vi "Save.vi"(0 "Reporte IN":refnum<class "NI_report.lvclass">, 7 "Error IN":errorcluster, 8 "X1":dbl[](array[numeric]), 9 "X7":dbl[](array[numeric]), 10 "X2":dbl[](array[numeric]), 11 "X8":dbl[](array[numeric]), 12 "X3":dbl[](array[numeric]), 13 "X9":dbl[](array[numeric]), 14 "X4":dbl[](array[numeric]), 16 "X5":dbl[](array[numeric]), 18 "X6":dbl[](array[numeric])) -> (20 "Reporte Out":refnum<class "NI_report.lvclass">, 27 "ERROR OUT":errorcluster)   [LabVIEW 2021]
uses:
  <vilib>/Utility/NIReport.llb/NI_report.lvclass
  <vilib>/addons/_office/excel.llb/Excel Easy Table (str).vi
  <vilib>/addons/_office/NI_ReportGenerationToolkit.lvlib
panel:
  out "XString 9":string[](array[string])
  out "XString 8":string[](array[string])
  out "XString 7":string[](array[string])
  out "XString 6":string[](array[string])
  out "XString 5":string[](array[string])
  out "XString 4":string[](array[string])
  out "XString 3":string[](array[string])
  out "XString 2":string[](array[string])
  out "XString":string[](array[string])
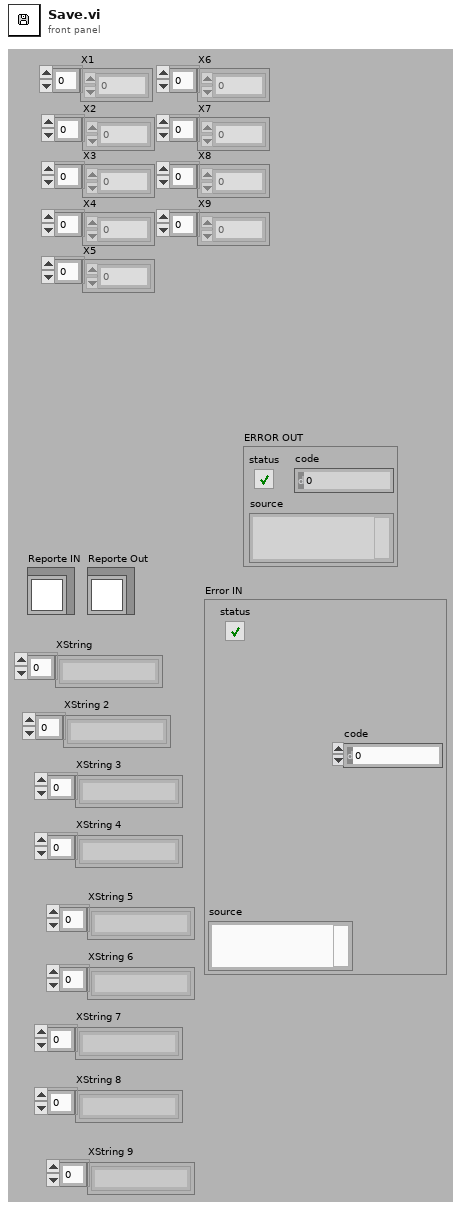
[diagram p1: front panel]
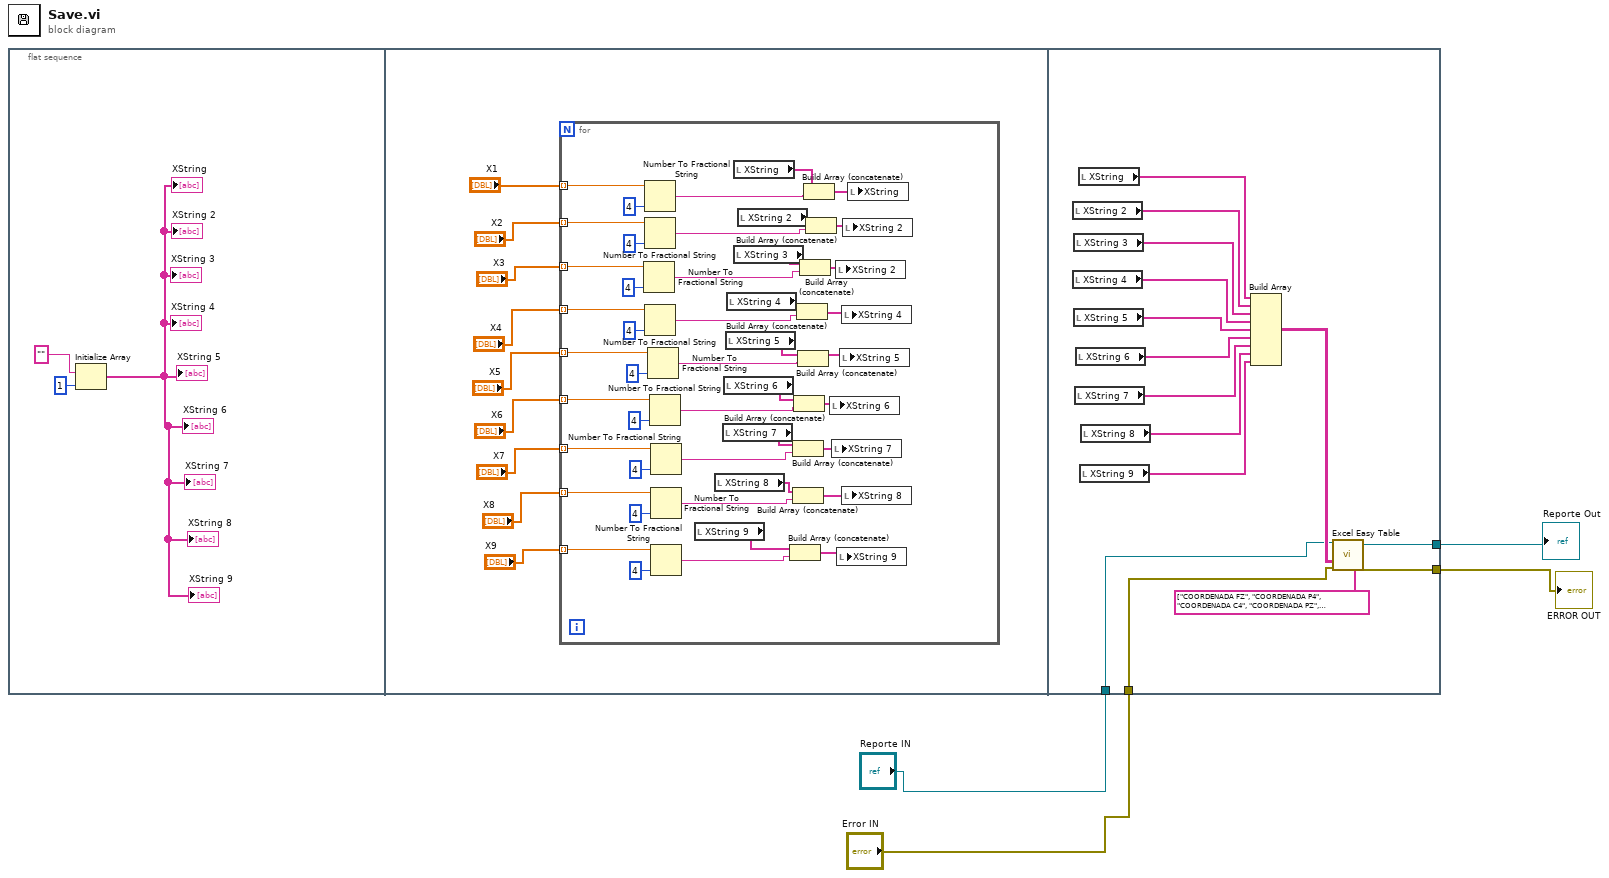
[diagram p0: block diagram]
diagram:
  n1 = flat-sequence {
    tunnel: "Reporte IN" -> [w65]
    tunnel: "Error IN" -> [w64]
    tunnel: [w63] -> w1
    tunnel: [w62] -> w2
    frame #0 {
      n2 = Initialize Array("", 1 ("dimension size")) -> (→"XString" →"XString 2" →"XString 3" →"XString 4" →"XString 5" →"XString 6" →"XString 7" →"XString 8" →"XString 9":string[])
    }
    frame #1 {
      n3 = for {
        tunnel: "X1" -> [w61] mode=indexing
        tunnel: "X2" -> [w51] mode=indexing
        tunnel: "X3" -> [w50] mode=indexing
        tunnel: "X4" -> [w49] mode=indexing
        tunnel: "X5" -> [w48] mode=indexing
        tunnel: "X6" -> [w47] mode=indexing
        tunnel: "X7" -> [w46] mode=indexing
        tunnel: "X8" -> [w45] mode=indexing
        tunnel: "X9" -> [w44] mode=indexing
        n4 = Number To Fractional String(number=w50, precision (6)=i16 4) -> (F-format string=w37:string)  [unwired: 2 in]
        n5 = Number To Fractional String(number=w61, precision (6)=i16 4) -> (F-format string=w43:string)  [unwired: 2 in]
        n6 = Number To Fractional String(number=w51, precision (6)=i16 4) -> (F-format string=w38:string)  [unwired: 2 in]
        n7 = Number To Fractional String(number=w49, precision (6)=i16 4) -> (F-format string=w34:string)  [unwired: 2 in]
        n8 = Number To Fractional String(number=w48, precision (6)=i16 4) -> (F-format string=w29:string)  [unwired: 2 in]
        n9 = Number To Fractional String(number=w47, precision (6)=i16 4) -> (F-format string=w27:string)  [unwired: 2 in]
        n10 = Number To Fractional String(number=w46, precision (6)=i16 4) -> (F-format string=w24:string)  [unwired: 2 in]
        n11 = Number To Fractional String(number=w45, precision (6)=i16 4) -> (F-format string=w22:string)  [unwired: 2 in]
        n12 = Number To Fractional String(number=w44, precision (6)=i16 4) -> (F-format string=w19:string)  [unwired: 2 in]
        n13 = local read "XString 9"() -> (w18:string[])
        n14 = local read "XString 8"() -> (w21:string[])
        n15 = local read "XString 7"() -> (w25:string[])
        n16 = local read "XString 6"() -> (w28:string[])
        n17 = local read "XString 5"() -> (w31:string[])
        n18 = local read "XString 4"() -> (w33:string[])
        n19 = local read "XString"() -> (w42:string[])
        n20 = local read "XString 3"() -> (w36:string[])
        n21 = local read "XString 2"() -> (w40:string[])
        n22 = Build Array (concatenate)(w18, w19) -> (w17:string[])
        n23 = Build Array (concatenate)(w25, w24) -> (w23:string[])
        n24 = Build Array (concatenate)(w21, w22) -> (w20:string[])
        n25 = Build Array (concatenate)(w28, w27) -> (w26:string[])
        n26 = Build Array (concatenate)(w33, w34) -> (w32:string[])
        n27 = Build Array (concatenate)(w31, w29) -> (w30:string[])
        n28 = Build Array (concatenate)(w36, w37) -> (w35:string[])
        n29 = Build Array (concatenate)(w42, w43) -> (w41:string[])
        n30 = Build Array (concatenate)(w40, w38) -> (w39:string[])
        n31 = local write "XString 6"(w26) -> ()
        n32 = local write "XString 7"(w23) -> ()
        n33 = local write "XString 2"(w35) -> ()
        n34 = local write "XString 9"(w17) -> ()
        n35 = local write "XString 5"(w30) -> ()
        n36 = local write "XString 4"(w32) -> ()
        n37 = local write "XString 8"(w20) -> ()
        n38 = local write "XString 2"(w39) -> ()
        n39 = local write "XString"(w41) -> ()
      }
    }
    frame #2 {
      n40 = local read "XString 2"() -> (w75:string[])
      n41 = local read "XString 4"() -> (w73:string[])
      n42 = local read "XString 3"() -> (w74:string[])
      n43 = local read "XString 5"() -> (w72:string[])
      n44 = local read "XString 7"() -> (w70:string[])
      n45 = local read "XString 6"() -> (w71:string[])
      n46 = local read "XString"() -> (w76:string[])
      n47 = local read "XString 9"() -> (w68:string[])
      n48 = local read "XString 8"() -> (w69:string[])
      n49 = Build Array(w76, w75, w74, w73, w72, w71, w70, w69, w68) -> (w67:string[][])
      n50 = call-poly <vilib>:"Excel Easy Table.vi"("report in"=w65, "text data"=w67, "error in (no error)"=w64, "column headers"=string[] ["COORDENADA FZ", "COORDENADA P4", "COORDENADA C4", "COORDENADA PZ", "COORDENADA F4", "COORDENADA C3", "COORDENADA P3", "COORDENADA F3", "COORDENADA CZ"]) -> ("report out"=w62:refnum<class "NI_report.lvclass">, "error out"=w63:errorcluster)  [unwired: 7 in, 3 out]
    }
  }
  "Reporte Out" <- w2
  "ERROR OUT" <- w1
